vi "Mouse Up.vi"(7 "Map Model in":refnum<class "Map Model.lvclass">, 8 "error in (no error)":errorcluster, 10 "Position":T1, 11 "Tool in":refnum<class "Tool.lvclass">) -> (0 "error out":errorcluster, 3 "Tool out":refnum<class "Tool.lvclass">, 5 "Map Model out":refnum<class "Map Model.lvclass">)   [LabVIEW 2020, in "Map Model.lvlib" / "Tool.lvclass"]
uses:
  Tool.lvclass
  <vilib>/Utility/miscctls.llb/LVPoint32TypeDef.ctl
  Map Model/Map Model.lvclass
  Tool.lvclass/Tool.ctl
  Map Model/Map Model.lvclass/Map Model.ctl
panel:
  # "NOTICE -- YOU MUST LEAVE THIS NOTICE IN PLACE.\n\nCopyright (c) 2017, LIANG LIU Shawn.Liu.cn@gmail.com\nAll rights reserved.\n\nRedistribution and use in source and binary forms, with or without modification, are permitted provided that the following conditions are met:\n-Redistributions of source code must retain the above copyright notice, this list of conditions and the following disclaimer.\n-Redistributions in binary form must reproduce the above copyright notice, this list of conditions and the following disclaimer in the documentation and/or other materials provided with the distribution.\n-Neither the name of the eLp nor the names of its contributors may be used to endorse or promote products derived from this software without specific prior written permission.\n\nTHIS SOFTWARE IS PROVIDED BY THE COPYRIGHT HOLDERS AND CONTRIBUTORS \"AS IS\" AND ANY EXPRESS OR IMPLIED WARRANTIES, INCLUDING, BUT NOT LIMITED TO, THE IMPLIED WARRANTIES OF MERCHANTABILITY AND FITNESS FOR A PARTICULAR PURPOSE ARE DISCLAIMED. IN NO EVENT SHALL THE COPYRIGHT HOLDER OR CONTRIBUTORS BE LIABLE FOR ANY DIRECT, INDIRECT, INCIDENTAL, SPECIAL, EXEMPLARY, OR CONSEQUENTIAL DAMAGES (INCLUDING, BUT NOT LIMITED TO, PROCUREMENT OF SUBSTITUTE GOODS OR SERVICES; LOSS OF USE, DATA, OR PROFITS; OR BUSINESS INTERRUPTION) HOWEVER CAUSED AND ON ANY THEORY OF LIABILITY, WHETHER IN CONTRACT, STRICT LIABILITY, OR TORT (INCLUDING NEGLIGENCE OR OTHERWISE) ARISING IN ANY WAY OUT OF THE USE OF THIS SOFTWARE, EVEN IF ADVISED OF THE POSSIBILITY OF SUCH DAMAGE."
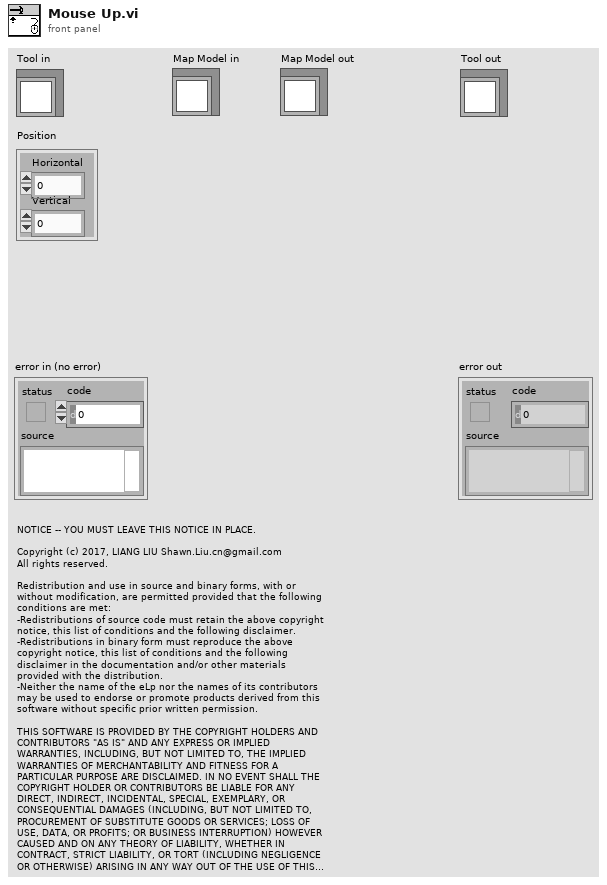
[diagram p1: front panel]
types:
  T1 = typedef "LVPoint32TypeDef.ctl" = cluster{"Horizontal":i32, "Vertical":i32}
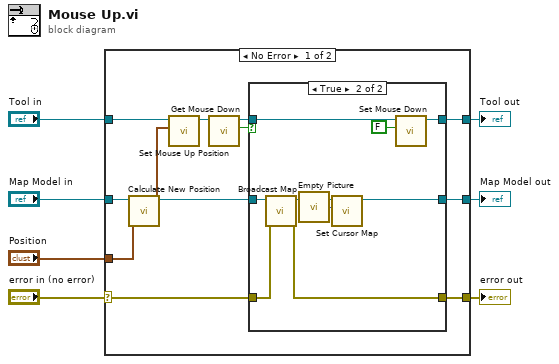
[diagram p0: block diagram]
diagram:
  n1 = case shown="No Error" "error in (no error)" {
    selector: "error in (no error)" -> [w14 w34]
    tunnel: "Tool in" -> [w19 w33]
    tunnel: [w18 w33] -> w6
    tunnel: "Map Model in" -> [w17 w32]
    tunnel: [w16 w34] -> w4
    tunnel: [w15 w32] -> w3
    tunnel: "Position" -> [w13 _]
    frame No Error {
      n2 = call "Calculate New Position.vi"("Position in"=w13, "Map Model in"=w17) -> ("Position out"=w8:T1, "Map Model out"=w9:refnum<class "Map Model.lvclass">)  [unwired: 8 in]
      n3 = call "Set Mouse Up Position.vi"("Mouse Up Position"=w8, "Tool in"=w19) -> ("Tool out"=w12:refnum<class "Tool.lvclass">)  [unwired: 9 in]
      n4 = call "Get Mouse Down.vi"("Tool in"=w12) -> ("Mouse Down"=w10:bool, "Tool out"=w11:refnum<class "Tool.lvclass">)  [unwired: 9 in]
      n5 = case shown="True" w10 {
        tunnel: [w22 w31] -> w18
        tunnel: w9 -> [w21 w24]
        tunnel: [w20 w30] -> w16
        tunnel: [w21 w25] -> w15
        tunnel: w11 -> [w22 w29]
        tunnel: w14 -> [w20 w23]
        frame False {
        }
        frame True {
          n6 = call "Broadcast Map.vi"("error in (no error)"=w23, "Map Model in"=w24) -> ("error out"=w30:errorcluster, "Map Model out"=w26:refnum<class "Map Model.lvclass">)  [unwired: 8 in]
          n7 = call "Empty Picture"() -> ("empty picture"=w27:picture)
          n8 = call "Set Cursor Map.vi"("Cursor Map"=w27, "Map Model in"=w26) -> ("Map Model out"=w25:refnum<class "Map Model.lvclass">)  [unwired: 9 in]
          n9 = call "Set Mouse Down.vi"("Mouse Down"=FALSE, "Tool in"=w29) -> ("Tool out"=w31:refnum<class "Tool.lvclass">)  [unwired: 9 in]
        }
      }
    }
    frame Error {
    }
  }
  "error out" <- w4
  "Tool out" <- w6
  "Map Model out" <- w3
